vi "Calibrate VNA.vi"(8 "error in (no error)":errorcluster, 9 "Cal kit type":enum16{"E-CAL", "Mechanical"}(ring), 10 "Calibration mode":enum16{"1 Port", "2  Port", "3 Port", "4 Port"}(ring), 11 "VNA-ZNB in":refnum<class "VNA-ZNB.lvclass">) -> (0 "error out":errorcluster, 3 "VNA-ZNB out":refnum<class "VNA-ZNB.lvclass">)   [LabVIEW 2020, in "VNA-ZNB.lvclass"]
uses:
  VNA-ZNB.lvclass
  C:/Sandbox/Git_Sandbox/WiSpry Test Framework source code (LV20)/WiSpry Test Framework/Instruments/Instrument.lvclass
  C:/Sandbox/Git_Sandbox/WiSpry Test Framework source code (LV20)/WiSpry Test Framework/Instruments/Vector Network Analyzer/Vector Network Analyzer.lvclass
  Vector Network Analyzer.lvclass/Vector Network Analyzer.ctl
  Instrument.lvclass/Instrument.ctl
  Instrument.lvclass
  Vector Network Analyzer.lvclass
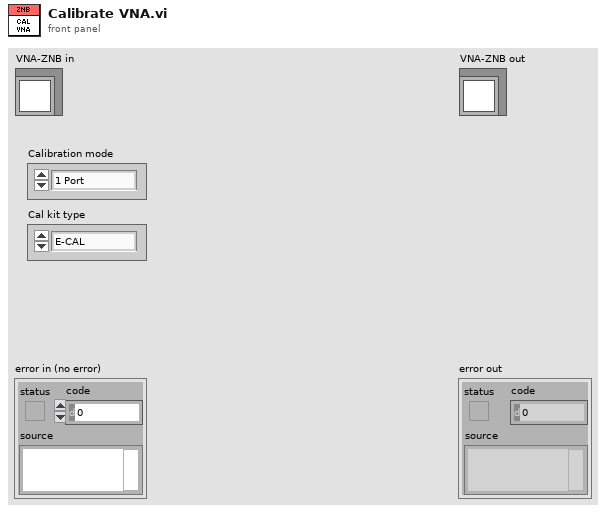
[diagram p1: front panel]
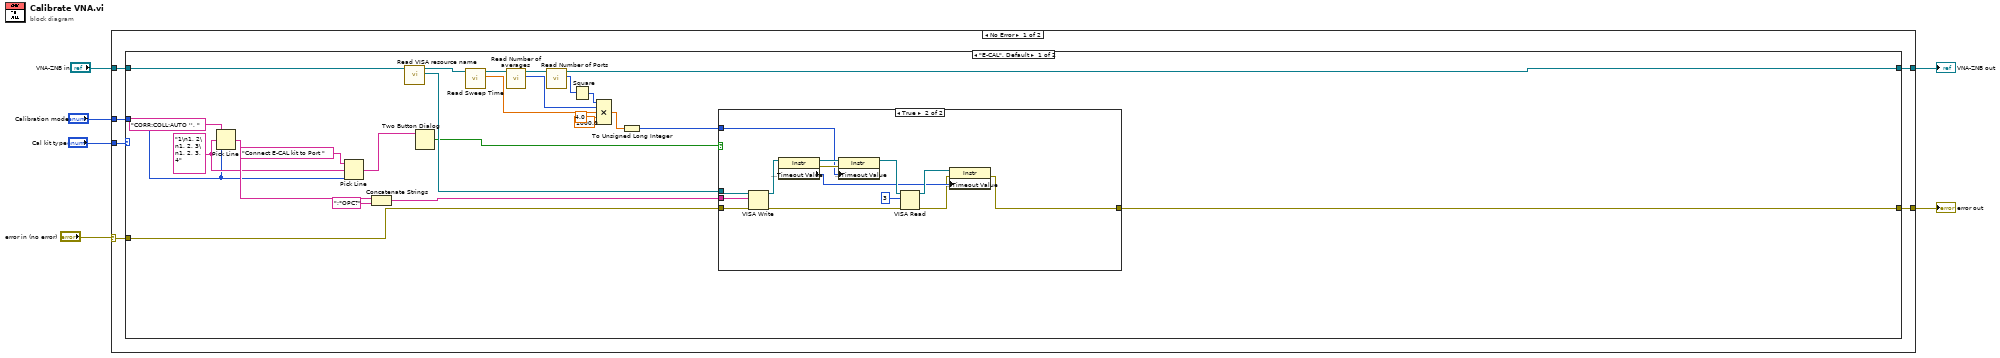
[diagram p0: block diagram]
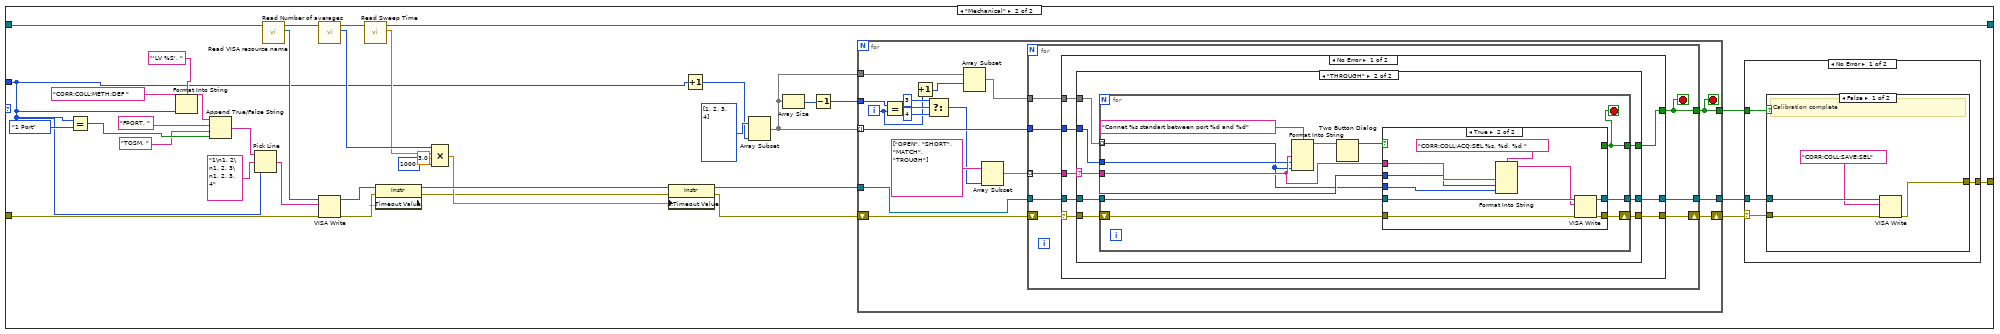
[diagram p3: hidden frame]
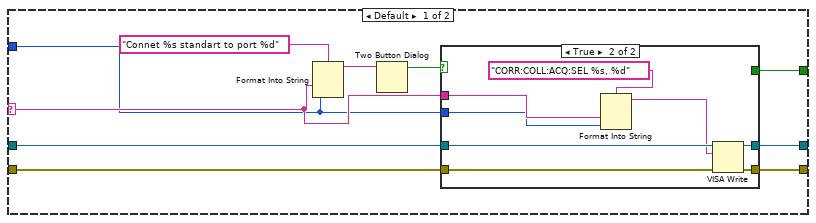
[diagram p6: hidden frame]
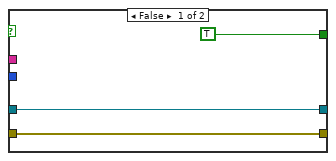
[diagram p7: hidden frame]
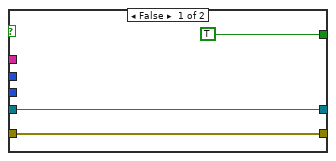
[diagram p8: hidden frame]
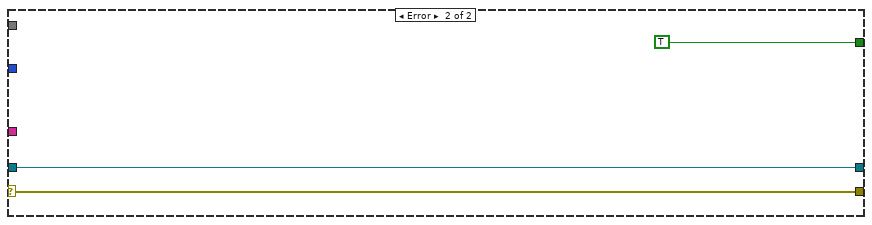
[diagram p9: hidden frame]
diagram:
  n1 = case shown="No Error" "error in (no error)" {
    selector: "error in (no error)" -> [w9 w188]
    tunnel: "Cal kit type" -> [w12 _]
    tunnel: "Calibration mode" -> [w11 _]
    tunnel: "VNA-ZNB in" -> [w10 w189]
    tunnel: [w8 w188] -> w2
    tunnel: [w7 w189] -> w1
    frame No Error {
      n2 = case shown="\"E-CAL\", Default" w12 {
        tunnel: w11 -> [w28 w53]
        tunnel: w10 -> [w36 w79]
        tunnel: w9 -> [w34 w80]
        tunnel: [w33 w54] -> w8
        tunnel: [w22 w60] -> w7
        frame "E-CAL", Default {
          w29 = "1\n1, 2\n1, 2, 3\n1, 2, 3, 4" ("multi-line string")
          n3 = Pick Line(string ("")="CORR:COLL:AUTO '', ", multi-line string=w29, line index=w28) -> (output string=w32:string)
          n4 = Pick Line(string ("")="Connect E-CAL kit to Port " ("message"), multi-line string=w29, line index=w28) -> (output string=w27:string)
          n5 = Concatenate Strings(w32, ";*OPC?" ("string")) -> (w26:string)
          n6 = call "Read VISA resource name.vi"("Instrument in"=w36) -> ("VISA resource name"=w35:refnum<visa-resource-name>, "Instrument out"=w24:refnum<class "VNA-ZNB.lvclass">)  [unwired: 9 in]
          n7 = Two Button Dialog(message=w27) -> (T button?=w31:bool)  [unwired: 2 in]
          n8 = call "Read Sweep Time.vi"("Vector Network Analyzer in"=w24) -> ("Sweep Time"=w17:dbl, "Vector Network Analyzer out"=w23:refnum<class "VNA-ZNB.lvclass">)  [unwired: 9 in]
          n9 = call "Read Number of averages.vi"("Vector Network Analyzer in"=w23) -> ("Number of averages"=w18:i32, "Vector Network Analyzer out"=w21:refnum<class "VNA-ZNB.lvclass">)  [unwired: 9 in]
          n10 = call "Read Number of Ports.vi"("Vector Network Analyzer in"=w21) -> ("Number of Ports"=w20:i32, "Vector Network Analyzer out"=w22:refnum<class "VNA-ZNB.lvclass">)  [unwired: 9 in]
          n11 = Square(x=w20) -> (x^2=w19:i32)
          n12 = Compound Arithmetic op=MULTIPLY(w19, w18, w17, 4.0 ("value"), 1000.0 ("value")) -> (w14:dbl)
          n13 = To Unsigned Long Integer(number=w14) -> (unsigned 32bit integer=w13:u32)
          n14 = case shown="True" w31 {
            tunnel: w35 -> [_ w52]
            tunnel: w34 -> [w38 w51]
            tunnel: [w38 w39] -> w33
            tunnel: w26 -> [_ w50]
            tunnel: w13 -> [_ w40]
            frame False {
            }
            frame True {
              n15 = VISA Write(VISA resource name=w52, write buffer=w50, error in (no error)=w51) -> (VISA resource name out=w49:refnum<visa-resource-name>, error out=w45:errorcluster)  [unwired: 1 out]
              n16 = property class="Instr"(reference=w49) -> (reference out=w48:refnum<visa-resource-name>, error out=w47:errorcluster, "General Settings:Timeout Value"=w42:u32)  [unwired: 1 in]
              n17 = property class="Instr"(reference=w48, error in=w47, "General Settings:Timeout Value"=w40) -> (reference out=w46:refnum<visa-resource-name>)  [unwired: 1 out]
              n18 = VISA Read(VISA resource name=w46, byte count=u32 3, error in (no error)=w45) -> (VISA resource name out=w43:refnum<visa-resource-name>, error out=w41:errorcluster)  [unwired: 2 out]
              n19 = property class="Instr"(reference=w43, error in=w41, "General Settings:Timeout Value"=w42) -> (error out=w39:errorcluster)  [unwired: 1 out]
            }
          }
        }
        frame "Mechanical" {
          n20 = Equal?(x=w53, y=enum16{"1 Port", "2  Port", "3 Port", "4 Port"}."1 Port") -> (x = y?=w88:bool)
          n21 = Format Into String(format string="'LV %S', ", initial string="CORR:COLL:METH:DEF ", w53) -> (resulting string=w83:string)  [unwired: 1 in, 1 out]
          n22 = Append True/False String(1:w88, 2:"TOSM, ", 3:"FPORT, ", 4:w83) -> (0:w82:string)
          n23 = Pick Line(string ("")=w82, multi-line string="1\n1, 2\n1, 2, 3\n1, 2, 3, 4", line index=w53) -> (output string=w77:string)
          n24 = call "Read VISA resource name.vi"("Instrument in"=w79) -> ("VISA resource name"=w78:refnum<visa-resource-name>, "Instrument out"=w72:refnum<class "VNA-ZNB.lvclass">)  [unwired: 9 in]
          n25 = call "Read Number of averages.vi"("Vector Network Analyzer in"=w72) -> ("Number of averages"=w70:i32, "Vector Network Analyzer out"=w71:refnum<class "VNA-ZNB.lvclass">)  [unwired: 9 in]
          n26 = VISA Write(VISA resource name=w78, write buffer=w77, error in (no error)=w80) -> (VISA resource name out=w68:refnum<visa-resource-name>, error out=w67:errorcluster)  [unwired: 1 out]
          n27 = call "Read Sweep Time.vi"("Vector Network Analyzer in"=w71) -> ("Sweep Time"=w69:dbl, "Vector Network Analyzer out"=w60:refnum<class "VNA-ZNB.lvclass">)  [unwired: 9 in]
          n28 = property class="Instr" props=["General Settings:Timeout Value"](reference=w68, error in=w67) -> (reference out=w66:refnum<visa-resource-name>, error out=w63:errorcluster)  [unwired: 1 out]
          n29 = Compound Arithmetic op=MULTIPLY(w70, w69, 3.0 ("value"), 1000 ("value")) -> (w64:dbl)
          n30 = property class="Instr"(reference=w66, error in=w63, "General Settings:Timeout Value"=w64) -> (reference out=w62:refnum<visa-resource-name>, error out=w61:errorcluster)
          n31 = Increment(x=w53) -> (x+1=w75:enum16{"1 Port", "2  Port", "3 Port", "4 Port"})
          n32 = Array Subset(array=i32[] [1, 2, 3, 4], length=w75) -> (w58:i32[])  [unwired: 1 in]
          n33 = Array Size(array=w58) -> (size(s)=w74:i32)
          n34 = Decrement(x=w74) -> (x-1=w73:i32)
          n35 = for {
            shift-right: [w102] -> w57
            shift-left: w61 -> [w110]
            tunnel: w58 -> [w109] mode=indexing
            tunnel: w73 -> [w116]
            tunnel: w62 -> [w108]
            tunnel: w58 -> [w106]
            tunnel: [w101] -> w56
            tunnel: [w100] -> w55
            i -> [w104]
            stop <- w101 stop-if-true
            n36 = Equal?(x=w116, y=w104) -> (x = y?=w114:bool)
            n37 = Increment(x=w104) -> (x+1=w105:i32)
            n38 = Select(t=3, s=w114, f=4) -> (s? t:f=w107:i32)
            n39 = Array Subset(array=w106, index=w105) -> (w103:i32[])  [unwired: 1 in]
            n40 = Array Subset(array=string[] ["OPEN", "SHORT", "MATCH", "TROUGH"], length=w107) -> (w111:string[])  [unwired: 1 in]
            n41 = for {
              tunnel: w111 -> [w122] mode=indexing
              shift-right: [w119] -> w102
              shift-left: w110 -> [w124]
              tunnel: [w123] -> w101
              tunnel: w108 -> [w121]
              tunnel: w109 -> [w120]
              tunnel: w103 -> [w118]
              tunnel: [w117] -> w100
              stop <- w123 stop-if-true
              n42 = case shown="No Error" w124 {
                selector: w124 -> [w131 w186]
                tunnel: [w128 TRUE] -> w123
                tunnel: w122 -> [w132 _]
                tunnel: w121 -> [w129 w185]
                tunnel: w120 -> [w130 _]
                tunnel: [w127 w186] -> w119
                tunnel: w118 -> [w126 _]
                tunnel: [w125 w185] -> w117
                frame No Error {
                  n43 = case shown="\"THROUGH\"" w132 {
                    selector: w132 -> [w137 w159]
                    tunnel: w131 -> [w139 w161]
                    tunnel: w130 -> [w136 w156]
                    tunnel: w129 -> [w138 w160]
                    tunnel: [w135 w158] -> w128
                    tunnel: [w134 w157] -> w127
                    tunnel: w126 -> [_ w155]
                    tunnel: [w133 w154] -> w125
                    frame Default {
                      n44 = Format Into String(format string="Connet %s standart to port %d", w137, w136) -> (resulting string=w141:string)  [unwired: 2 in, 1 out]
                      n45 = Two Button Dialog(message=w141) -> (T button?=w140:bool)  [unwired: 2 in]
                      n46 = case shown="True" w140 {
                        tunnel: w139 -> [w144 w150]
                        tunnel: w138 -> [w143 w149]
                        tunnel: w137 -> [_ w152]
                        tunnel: w136 -> [_ w151]
                        tunnel: [TRUE _] -> w135
                        tunnel: [w144 w147] -> w134
                        tunnel: [w143 w146] -> w133
                        frame False {
                        }
                        frame True {
                          n47 = Format Into String(format string="CORR:COLL:ACQ:SEL %s, %d", w152, w151) -> (resulting string=w148:string)  [unwired: 2 in, 1 out]
                          n48 = VISA Write(VISA resource name=w149, write buffer=w148, error in (no error)=w150) -> (VISA resource name out=w146:refnum<visa-resource-name>, error out=w147:errorcluster)  [unwired: 1 out]
                        }
                      }
                    }
                    frame "THROUGH" {
                      n49 = for {
                        tunnel: w160 -> [w168]
                        tunnel: w159 -> [w167]
                        tunnel: [w164] -> w158
                        tunnel: w156 -> [w165]
                        shift-right: [w166] -> w157
                        shift-left: w161 -> [w169]
                        tunnel: w155 -> [w163] mode=indexing
                        tunnel: [w162] -> w154
                        stop <- w164 stop-if-true
                        n50 = Format Into String(format string="Connet %s standart between port %d and %d", w167, w165, w163) -> (resulting string=w171:string)  [unwired: 2 in, 1 out]
                        n51 = Two Button Dialog(message=w171) -> (T button?=w170:bool)  [unwired: 2 in]
                        n52 = case shown="True" w170 {
                          tunnel: w169 -> [w174 w181]
                          tunnel: w168 -> [w173 w180]
                          tunnel: w167 -> [_ w183]
                          tunnel: w165 -> [_ w182]
                          tunnel: [TRUE _] -> w164
                          tunnel: [w174 w178] -> w166
                          tunnel: w163 -> [_ w177]
                          tunnel: [w173 w176] -> w162
                          frame False {
                          }
                          frame True {
                            n53 = Format Into String(format string="CORR:COLL:ACQ:SEL %s, %d, %d ", w183, w182, w177) -> (resulting string=w179:string)  [unwired: 2 in, 1 out]
                            n54 = VISA Write(VISA resource name=w180, write buffer=w179, error in (no error)=w181) -> (VISA resource name out=w176:refnum<visa-resource-name>, error out=w178:errorcluster)  [unwired: 1 out]
                          }
                        }
                      }
                    }
                  }
                }
                frame Error {
                }
              }
            }
          }
          n55 = case shown="No Error" w57 {
            selector: w57 -> [w92 w99]
            tunnel: w56 -> [w93 _]
            tunnel: w55 -> [w91 _]
            tunnel: [w90 w99] -> w54
            frame No Error {
              n56 = case shown="False" w93 {
                tunnel: w92 -> [w97 w98]
                tunnel: w91 -> [w96 _]
                tunnel: [w95 w98] -> w90
                frame False {
                  # "Calibration complete"
                  n57 = VISA Write(VISA resource name=w96, write buffer="CORR:COLL:SAVE:SEL", error in (no error)=w97) -> (error out=w95:errorcluster)  [unwired: 2 out]
                }
                frame True {
                }
              }
            }
            frame Error {
            }
          }
        }
      }
    }
    frame Error {
    }
  }
  "error out" <- w2
  "VNA-ZNB out" <- w1
